vi "Check Types.vi"(7 "Name Root":string, 8 "error in (no error)":errorcluster, 11 "Variant":variant) -> (0 "error out":errorcluster)   [LabVIEW 2021, in "BT.lvlib" / "bt_Send_Synch_WithValues.lvclass"]
uses:
  Blackboard/Blackboard.lvclass/Blackboard.ctl
  <vilib>/TSA/Omni-Bus/Local Bus/Support/DBL/Local Bus_DBL.lvclass
  C:/Program Files (x86)/National Instruments/LabVIEW 2021/vi.lib/TSA/Abstract Data Classes/Abs_Types/Value/Abs_Value.lvclass
  <vilib>/TSA/Omni-Bus/Local Bus/Support/SGL/Local Bus_SGL.lvclass
  <vilib>/TSA/Omni-Bus/Local Bus/Support/EXT/Local Bus_EXT.lvclass
  <vilib>/TSA/Omni-Bus/Local Bus/Support/Bool/Local Bus_Boolean.lvclass
  <vilib>/TSA/Omni-Bus/Local Bus/Support/STR/Local Bus_String.lvclass
  <vilib>/TSA/Omni-Bus/Local Bus/Support/Variant/Local Bus_Variant.lvclass
  <vilib>/TSA/Omni-Bus/Local Bus/Support/WFM/Local Bus_Waveform.lvclass
  <vilib>/TSA/Omni-Bus/Local Bus/Support/Time/Local Bus_Time.lvclass
  <vilib>/TSA/Omni-Bus/Local Bus/Support/U8/Local Bus_U8.lvclass
  <vilib>/TSA/Omni-Bus/Local Bus/Support/U16/Local Bus_U16.lvclass
  <vilib>/TSA/Omni-Bus/Local Bus/Support/U32/Local Bus_U32.lvclass
  <vilib>/TSA/Omni-Bus/Local Bus/Support/U64/Local Bus_U64.lvclass
  <vilib>/TSA/Omni-Bus/Local Bus/Support/I8/Local Bus_I8.lvclass
  <vilib>/TSA/Omni-Bus/Local Bus/Support/I16/Local Bus_I16.lvclass
  <vilib>/TSA/Omni-Bus/Local Bus/Support/I32/Local Bus_I32.lvclass
  <vilib>/TSA/Omni-Bus/Local Bus/Support/I64/Local Bus_I64.lvclass
  <vilib>/TSA/Omni-Bus/Local Bus/Support/CSGL/Local Bus_CSGL.lvclass
  <vilib>/TSA/Omni-Bus/Local Bus/Support/CDBL/Local Bus_CDBL.lvclass
  <vilib>/TSA/Omni-Bus/Local Bus/Support/CEXT/Local Bus_CEXT.lvclass
  <vilib>/TSA/Omni-Bus/Local Bus/Support/Type/Local Bus_Type.lvclass
  <vilib>/TSA/Abstract Data Classes/Abs_Types/Type/Abs_Type.lvclass
  <vilib>/Utility/error.llb/Error Cluster From Error Code.vi
  bt_Send_Synch_WithValues.lvclass
  bt_Send_Synch_WithValues.lvclass/bt_Send_Synch_WithValues.ctl
  <vilib>/Utility/Data Type/NI_Data Type.lvlib
  <vilib>/ErrorRing/Error Ring.xnode
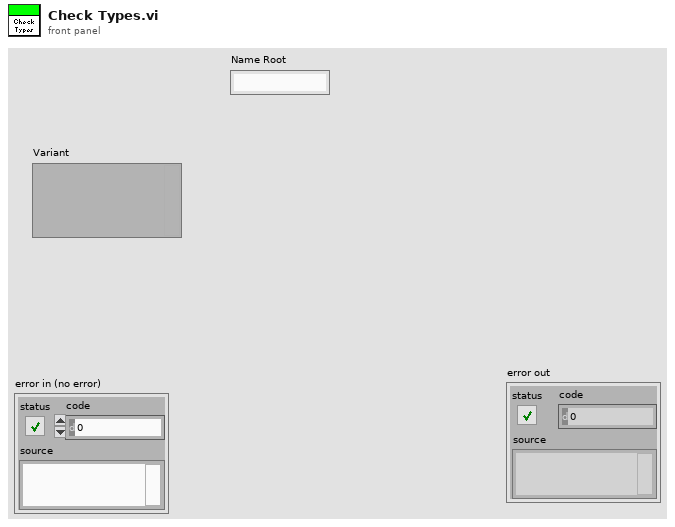
[diagram p1: front panel]
types:
  T1 = typedef "NI_Data Type.lvlib/Data Type.ctl" = enum8{"Invalid Type", "Void", "I8", "I16", "I32", "I64", "U8", "U16", "U32", "U64", "Single Float", "Double Float", "Extended Float", "Single Complex", "Double Complex", "Extended Complex", "Enum U8", "Enum U16", "Enum U32", "Enum U64", "Single Float With Unit", "Double Float With Unit", "Extended Float With Unit", "Single Complex with Unit", "Double Complex with Unit", "Extended Complex with Unit", "Boolean", "String", "Path", "Picture", "Tag", "Array", "Cluster", "Variant", "LV Variant", "Waveform", "Timestamp", "Digital Waveform", "Digital Data", "ExpressData", "Refnum", "External Data", "VI", "Poly VI", "LabVIEW Class Instance", "Fixed Point", "Set Collection", "Map Collection"}
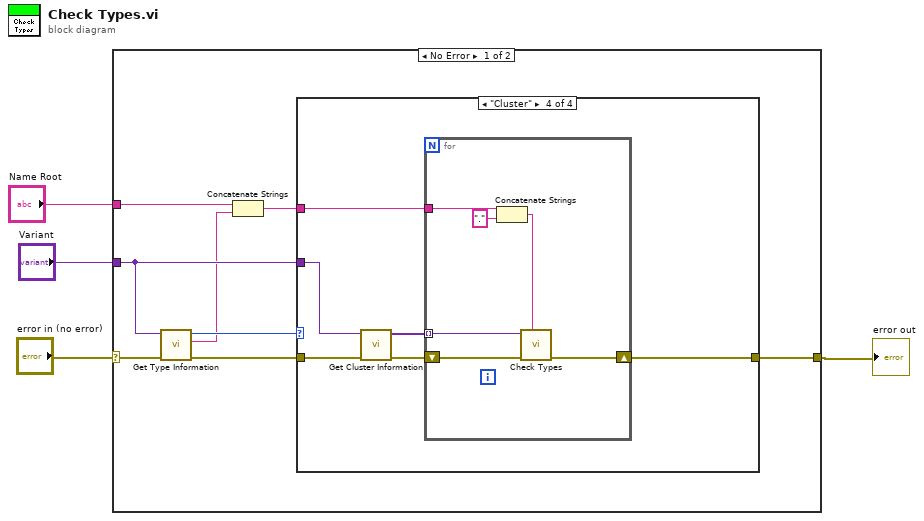
[diagram p0: block diagram]
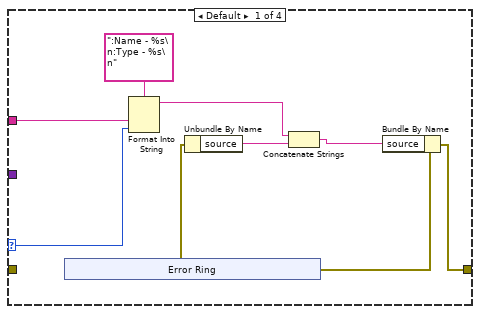
[diagram p2: hidden frame]
diagram:
  n1 = case shown="No Error" "error in (no error)" {
    selector: "error in (no error)" -> [w12 w39]
    tunnel: "Variant" -> [w9 _]
    tunnel: "Name Root" -> [w6 _]
    tunnel: [w5 w39] -> w1
    frame No Error {
      n2 = call <vilib>:"Get Type Information.vi"("error in (no error)"=w12, "variant"=w9) -> ("error out"=w10:errorcluster, "name"=w7:string, "type"=w11:T1)  [unwired: 5 in, 2 out]
      n3 = Concatenate Strings(w6, w7) -> (w8:string)
      n4 = case shown="\"Cluster\"" w11 {
        selector: w11 -> [w13 _ _ _]
        tunnel: w10 -> [_ w25 w26 w32]
        tunnel: w9 -> [_ _ _ w31]
        tunnel: [w20 w25 w26 w28] -> w5
        tunnel: w8 -> [w14 _ _ w27]
        frame Default {
          n5 = xnode "Error Ring"() -> ("error out"=w19:errorcluster)
          n6 = Format Into String(format string=":Name - %s\n:Type - %s\n", w14, w13) -> (resulting string=w15:string)  [unwired: 2 in, 1 out]
          n7 = Unbundle By Name(w19) -> ("source"=w18:string)
          n8 = Concatenate Strings(w15, w18) -> (w17:string)
          n9 = Bundle By Name(cluster=w19, "source"=w17) -> (w20:errorcluster)
        }
        frame "I8".."Extended Complex", "Boolean", "String", "Variant".."Timestamp" {
        }
        frame "Enum U8".."Enum U64" {
        }
        frame "Cluster" {
          n10 = call <vilib>:"Get Cluster Information.vi"("error in (no error)"=w32, "variant"=w31) -> ("error out"=w30:errorcluster, "cluster elements"=w29:variant[])  [unwired: 8 in]
          n11 = for {
            tunnel: w29 -> [w33] mode=indexing
            shift-right: [w37] -> w28
            shift-left: w30 -> [w38]
            tunnel: w27 -> [w36]
            n12 = Concatenate Strings(w36, "." ("string")) -> (w34:string)
            n13 = call "Check Types.vi"("Name Root"=w34, "error in (no error)"=w38, "Variant"=w33) -> ("error out"=w37:errorcluster)  [unwired: 8 in]
          }
        }
      }
    }
    frame Error {
    }
  }
  "error out" <- w1
